vi "test-path-planner-basic.vi"() -> ()   [LabVIEW 2019]
uses:
  <vilib>/Rock Robotics/WPI/ThirdParty/MJansen/PathPlanner/PathPlannerTrajectory.ctl
  <vilib>/Rock Robotics/WPI/ThirdParty/MJansen/PathPlanner/PathPlannerState.ctl
  <vilib>/Rock Robotics/WPI/ThirdParty/JAS_Junk/TrajLib/TypeDef/ROTATION2D.ctl
  <vilib>/Rock Robotics/WPI/ThirdParty/JAS_Junk/TrajLib/TypeDef/TRAJ_STATE.ctl
  <vilib>/Rock Robotics/WPI/ThirdParty/JAS_Junk/TrajLib/TypeDef/POSE2D.ctl
  <vilib>/Rock Robotics/WPI/ThirdParty/JAS_Junk/TrajLib/TypeDef/TRANSLATION2D.ctl
  <vilib>/Rock Robotics/WPI/ThirdParty/MJansen/PathPlanner/PathPlannerWaypoint.ctl
  <vilib>/Rock Robotics/WPI/ThirdParty/JAS_Junk/TrajLib/Util_ApproxEquals.vi
  <vilib>/Rock Robotics/WPI/ThirdParty/JAS_Junk/TrajLib/TrajectoryState_Equals.vi
  <vilib>/Rock Robotics/WPI/ThirdParty/JAS_Junk/TrajLib/Pose2d_Equals.vi
  <vilib>/Rock Robotics/WPI/ThirdParty/JAS_Junk/TrajLib/Translation2d_Equals.vi
  <vilib>/Rock Robotics/WPI/ThirdParty/JAS_Junk/TrajLib/Rotation2d_Equals.vi
  <vilib>/Rock Robotics/WPI/ThirdParty/JAS_Junk/TrajLib/Util_CalcDist.vi
  <vilib>/Rock Robotics/WPI/ThirdParty/MJansen/PathPlanner/PathPlanner.lvlib
  <vilib>/Rock Robotics/WPI/ThirdParty/JAS_Junk/TrajLib/Trajectory_Library.lvlib
  <vilib>/Analysis/NI_AALBase.lvlib
panel:
  in  "Tab Control":T1(tab)
  in  "jsonReadTrajFile":string="C:\\Shares\\github\\PathPlannerLabVIEW\\PathPlannerSandbox\\PathPlannerTestPath\\Javapath1.json"
  in  "Max Velocity":dbl=3.0
  in  "Max Acceleration":dbl=2.0
  in  "stop":bool
  in  "Reversed":bool
  out "PathPlannerWayPoints":T2[](array[typedef]) {"HolonomicRotation"."SIN" format="%13.4f"; "HolonomicRotation"."COS" format="%13.4f"; "HolonomicRotation"."VALUE" format="%13.4f"; "NextControl"."Y" format="%14.3f"; "NextControl"."X" format="%14.3f"; "PrevControl"."Y" format="%14.3f"; "PrevControl"."X" format="%14.3f"; "AnchorPoint"."Y" format="%14.3f"; "AnchorPoint"."X" format="%14.3f"}
  in  "Path FileName":string="C:\\Shares\\github\\PathPlannerLabVIEW\\PathPlannerSandbox\\PathPlannerTestPath\\path1.path"
  out "LabVIEW path json read error":errorcluster
  in  "LabVIEW jsonWriteFile":string="C:\\Shares\\github\\PathPlannerLabVIEW\\PathPlannerSandbox\\PathPlannerTestPath\\LabVIEWpath1.json"
  out "Java File Read Error":errorcluster
  out "LabView Write\nJSON Error":errorcluster
  out "PathPlannerTrajectory":T5 {"States"."HolonomicAngular\nvelocity Deg/Sec"."SIN" format="%13.4f"; "States"."HolonomicAngular\nvelocity Deg/Sec"."COS" format="%13.4f"; "States"."HolonomicAngular\nvelocity Deg/Sec"."VALUE" format="%13.4f"; "States"."HolonomicRotation"."SIN" format="%13.4f"; "States"."HolonomicRotation"."COS" format="%13.4f"; "States"."HolonomicRotation"."VALUE" format="%13.4f"; "States"."AngularVelocity"."SIN" format="%13.4f"; "States"."AngularVelocity"."COS" format="%13.4f"; "States"."AngularVelocity"."VALUE" format="%13.4f"; "States"."TrajectoryState"."POSE"."ROTATION"."SIN" format="%13.4f"; "States"."TrajectoryState"."POSE"."ROTATION"."COS" format="%13.4f"; "States"."TrajectoryState"."POSE"."ROTATION"."VALUE" format="%13.4f"; "States"."TrajectoryState"."POSE"."TRANSLATION"."Y" format="%14.3f"; "States"."TrajectoryState"."POSE"."TRANSLATION"."X" format="%14.3f"; "States"."AngularAcceleration"."SIN" format="%13.4f"; "States"."AngularAcceleration"."COS" format="%13.4f"; "States"."AngularAcceleration"."VALUE" format="%13.4f"}
  out "outPathPlannerStates":T6[](array[typedef]) {"HolonomicAngular\nvelocity Deg/Sec"."SIN" format="%13.4f"; "HolonomicAngular\nvelocity Deg/Sec"."COS" format="%13.4f"; "HolonomicAngular\nvelocity Deg/Sec"."VALUE" format="%13.4f"; "HolonomicRotation"."SIN" format="%13.4f"; "HolonomicRotation"."COS" format="%13.4f"; "HolonomicRotation"."VALUE" format="%13.4f"; "AngularVelocity"."SIN" format="%13.4f"; "AngularVelocity"."COS" format="%13.4f"; "AngularVelocity"."VALUE" format="%13.4f"; "TrajectoryState"."POSE"."ROTATION"."SIN" format="%13.4f"; "TrajectoryState"."POSE"."ROTATION"."COS" format="%13.4f"; "TrajectoryState"."POSE"."ROTATION"."VALUE" format="%13.4f"; "TrajectoryState"."POSE"."TRANSLATION"."Y" format="%14.3f"; "TrajectoryState"."POSE"."TRANSLATION"."X" format="%14.3f"; "AngularAcceleration"."SIN" format="%13.4f"; "AngularAcceleration"."COS" format="%13.4f"; "AngularAcceleration"."VALUE" format="%13.4f"}
  in  "Down Button":bool
  in  "Up Button":bool
  in  "index":i32 step=20
  out "Java_TotalTime_Sec":dbl
  out "LabVIEW_TotalTime_Sec":dbl
  out "Jave and LabVIEW \nexactly equal":bool
  out "JavaStateCount":i32
  out "LabVIEWStateCount":i32
  out "States Check":bool[](array[boolean])
  out "JavaStates":T7[](array[typedef]) {"POSE"."ROTATION"."SIN" format="%13.4f"; "POSE"."ROTATION"."COS" format="%13.4f"; "POSE"."ROTATION"."VALUE" format="%13.4f"; "POSE"."TRANSLATION"."Y" format="%14.3f"; "POSE"."TRANSLATION"."X" format="%14.3f"}
  out "LabVIEWStates":T7[](array[typedef]) {"POSE"."ROTATION"."SIN" format="%13.4f"; "POSE"."ROTATION"."COS" format="%13.4f"; "POSE"."ROTATION"."VALUE" format="%13.4f"; "POSE"."TRANSLATION"."Y" format="%14.3f"; "POSE"."TRANSLATION"."X" format="%14.3f"}
  out "Differences":T7[](array[typedef]) {"POSE"."ROTATION"."SIN" format="%13.4f"; "POSE"."ROTATION"."COS" format="%13.4f"; "POSE"."ROTATION"."VALUE" format="%13.4f"; "POSE"."TRANSLATION"."Y" format="%14.3f"; "POSE"."TRANSLATION"."X" format="%14.3f"}
  out "max time diff":dbl
  out "max vel diff":dbl
  out "max accel diff":dbl
  out "max x diff":dbl
  out "max y diff":dbl
  out "max rot diff rad":dbl
  out "max curvature diff":dbl
  out "vel mean":dbl format="%0.6f"
  out "vel std dev":dbl format="%0.6f"
  out "accel mean":dbl format="%0.6f"
  out "accel std dev":dbl format="%0.6f"
  out "Java and LabVIEW \nwithin tolerance":bool
  in  "Tolerance":T7={"TimeSeconds"=0.15, "Velocity"=0.25, "Acceleration"=2.5, "POSE"={"TRANSLATION"={"X"=0.015, "Y"=0.015}, "ROTATION"={"VALUE"=0.01, "COS"=0.0, "SIN"=0.0}}, "Curvature"=1.4} {"POSE"."ROTATION"."SIN" format="%13.4f"; "POSE"."ROTATION"."COS" format="%13.4f"; "POSE"."ROTATION"."VALUE" format="%13.4f"; "POSE"."TRANSLATION"."Y" format="%14.3f"; "POSE"."TRANSLATION"."X" format="%14.3f"}
  out "XY SPLINE":cluster{dbl[], dbl[]}[](graph)
  out "XY Graph":cluster{dbl[], dbl[]}[](graph)
  out "Sample Graph":dbl[][](graph)
  out "LabVIEW Time Plot":cluster{dbl[], dbl[]}[](graph)
  out "Java Time Plot":cluster{dbl[], dbl[]}[](graph)
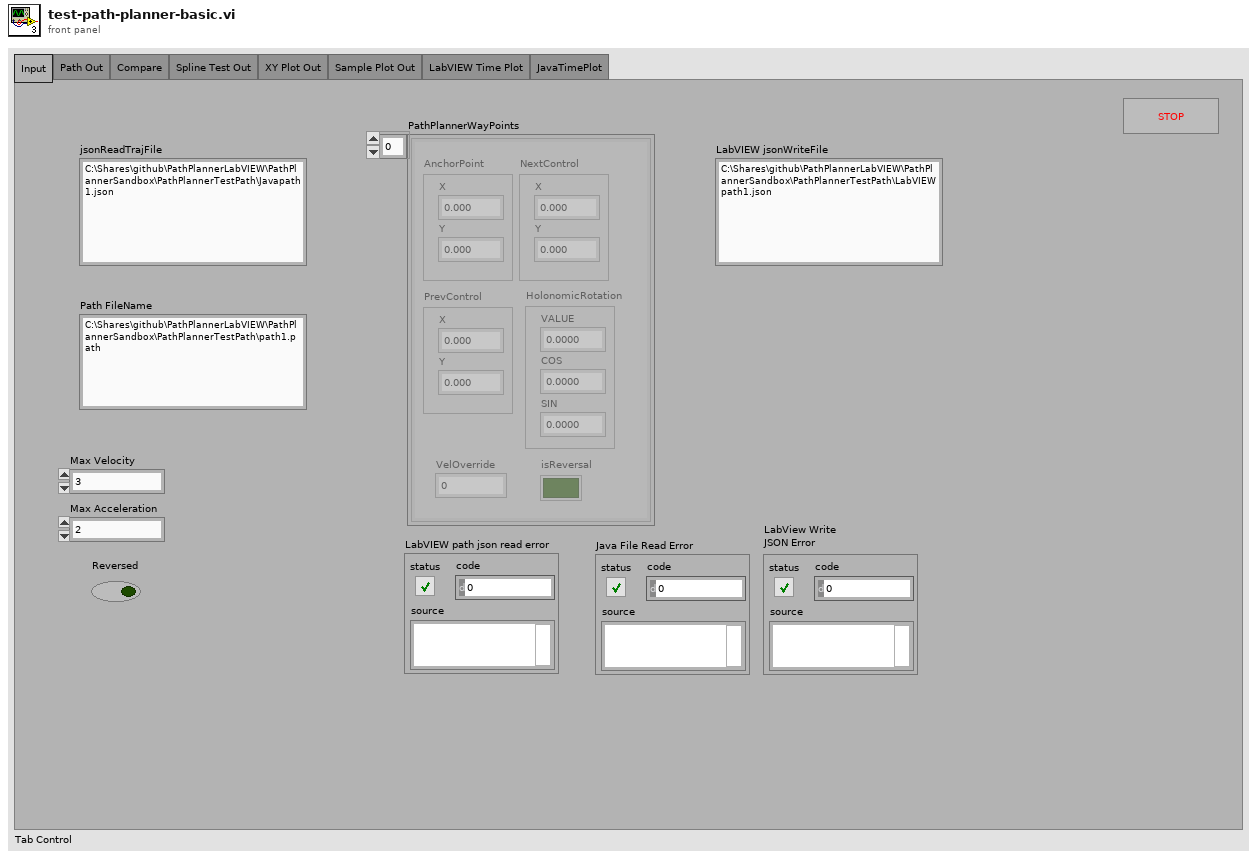
[diagram p1: front panel]
types:
  T1 = enum32{"Input", "Path Out", "Compare", "Spline Test Out", "XY Plot Out", "Sample Plot Out", "LabVIEW Time Plot", "JavaTimePlot"}
  T2 = typedef "PathPlanner.lvlib/PathPlannerWaypoint.ctl" = cluster{"AnchorPoint":T3, "PrevControl":T3, "NextControl":T3, "HolonomicRotation":T4, "VelOverride":dbl, "isReversal":bool}
  T3 = typedef "Trajectory_Library.lvlib/TRANSLATION2D.ctl" = cluster{"X":dbl, "Y":dbl}
  T4 = typedef "Trajectory_Library.lvlib/ROTATION2D.ctl" = cluster{"VALUE":dbl, "COS":dbl, "SIN":dbl}
  T5 = typedef "PathPlanner.lvlib/PathPlannerTrajectory.ctl" = cluster{"TotalTimeSeconds":dbl, "States":T6[]}
  T6 = typedef "PathPlanner.lvlib/PathPlannerState.ctl" = cluster{"AngularAcceleration":T4, "PositionMeters":dbl, "TrajectoryState":T7, "AngularVelocity":T4, "HolonomicRotation":T4, "CurveRadius":dbl, "DeltaPos":dbl, "HolonomicAngular\nvelocity Deg/Sec":T4}
  T7 = typedef "Trajectory_Library.lvlib/TRAJ_STATE.ctl" = cluster{"TimeSeconds":dbl, "Velocity":dbl, "Acceleration":dbl, "POSE":T8, "Curvature":dbl}
  T8 = typedef "Trajectory_Library.lvlib/POSE2D.ctl" = cluster{"TRANSLATION":T3, "ROTATION":T4}
  T9 = typedef "Trajectory_Library.lvlib/TRAJECTORY.ctl" = cluster{"TotalTImeSecs":dbl, "States":T7[]}
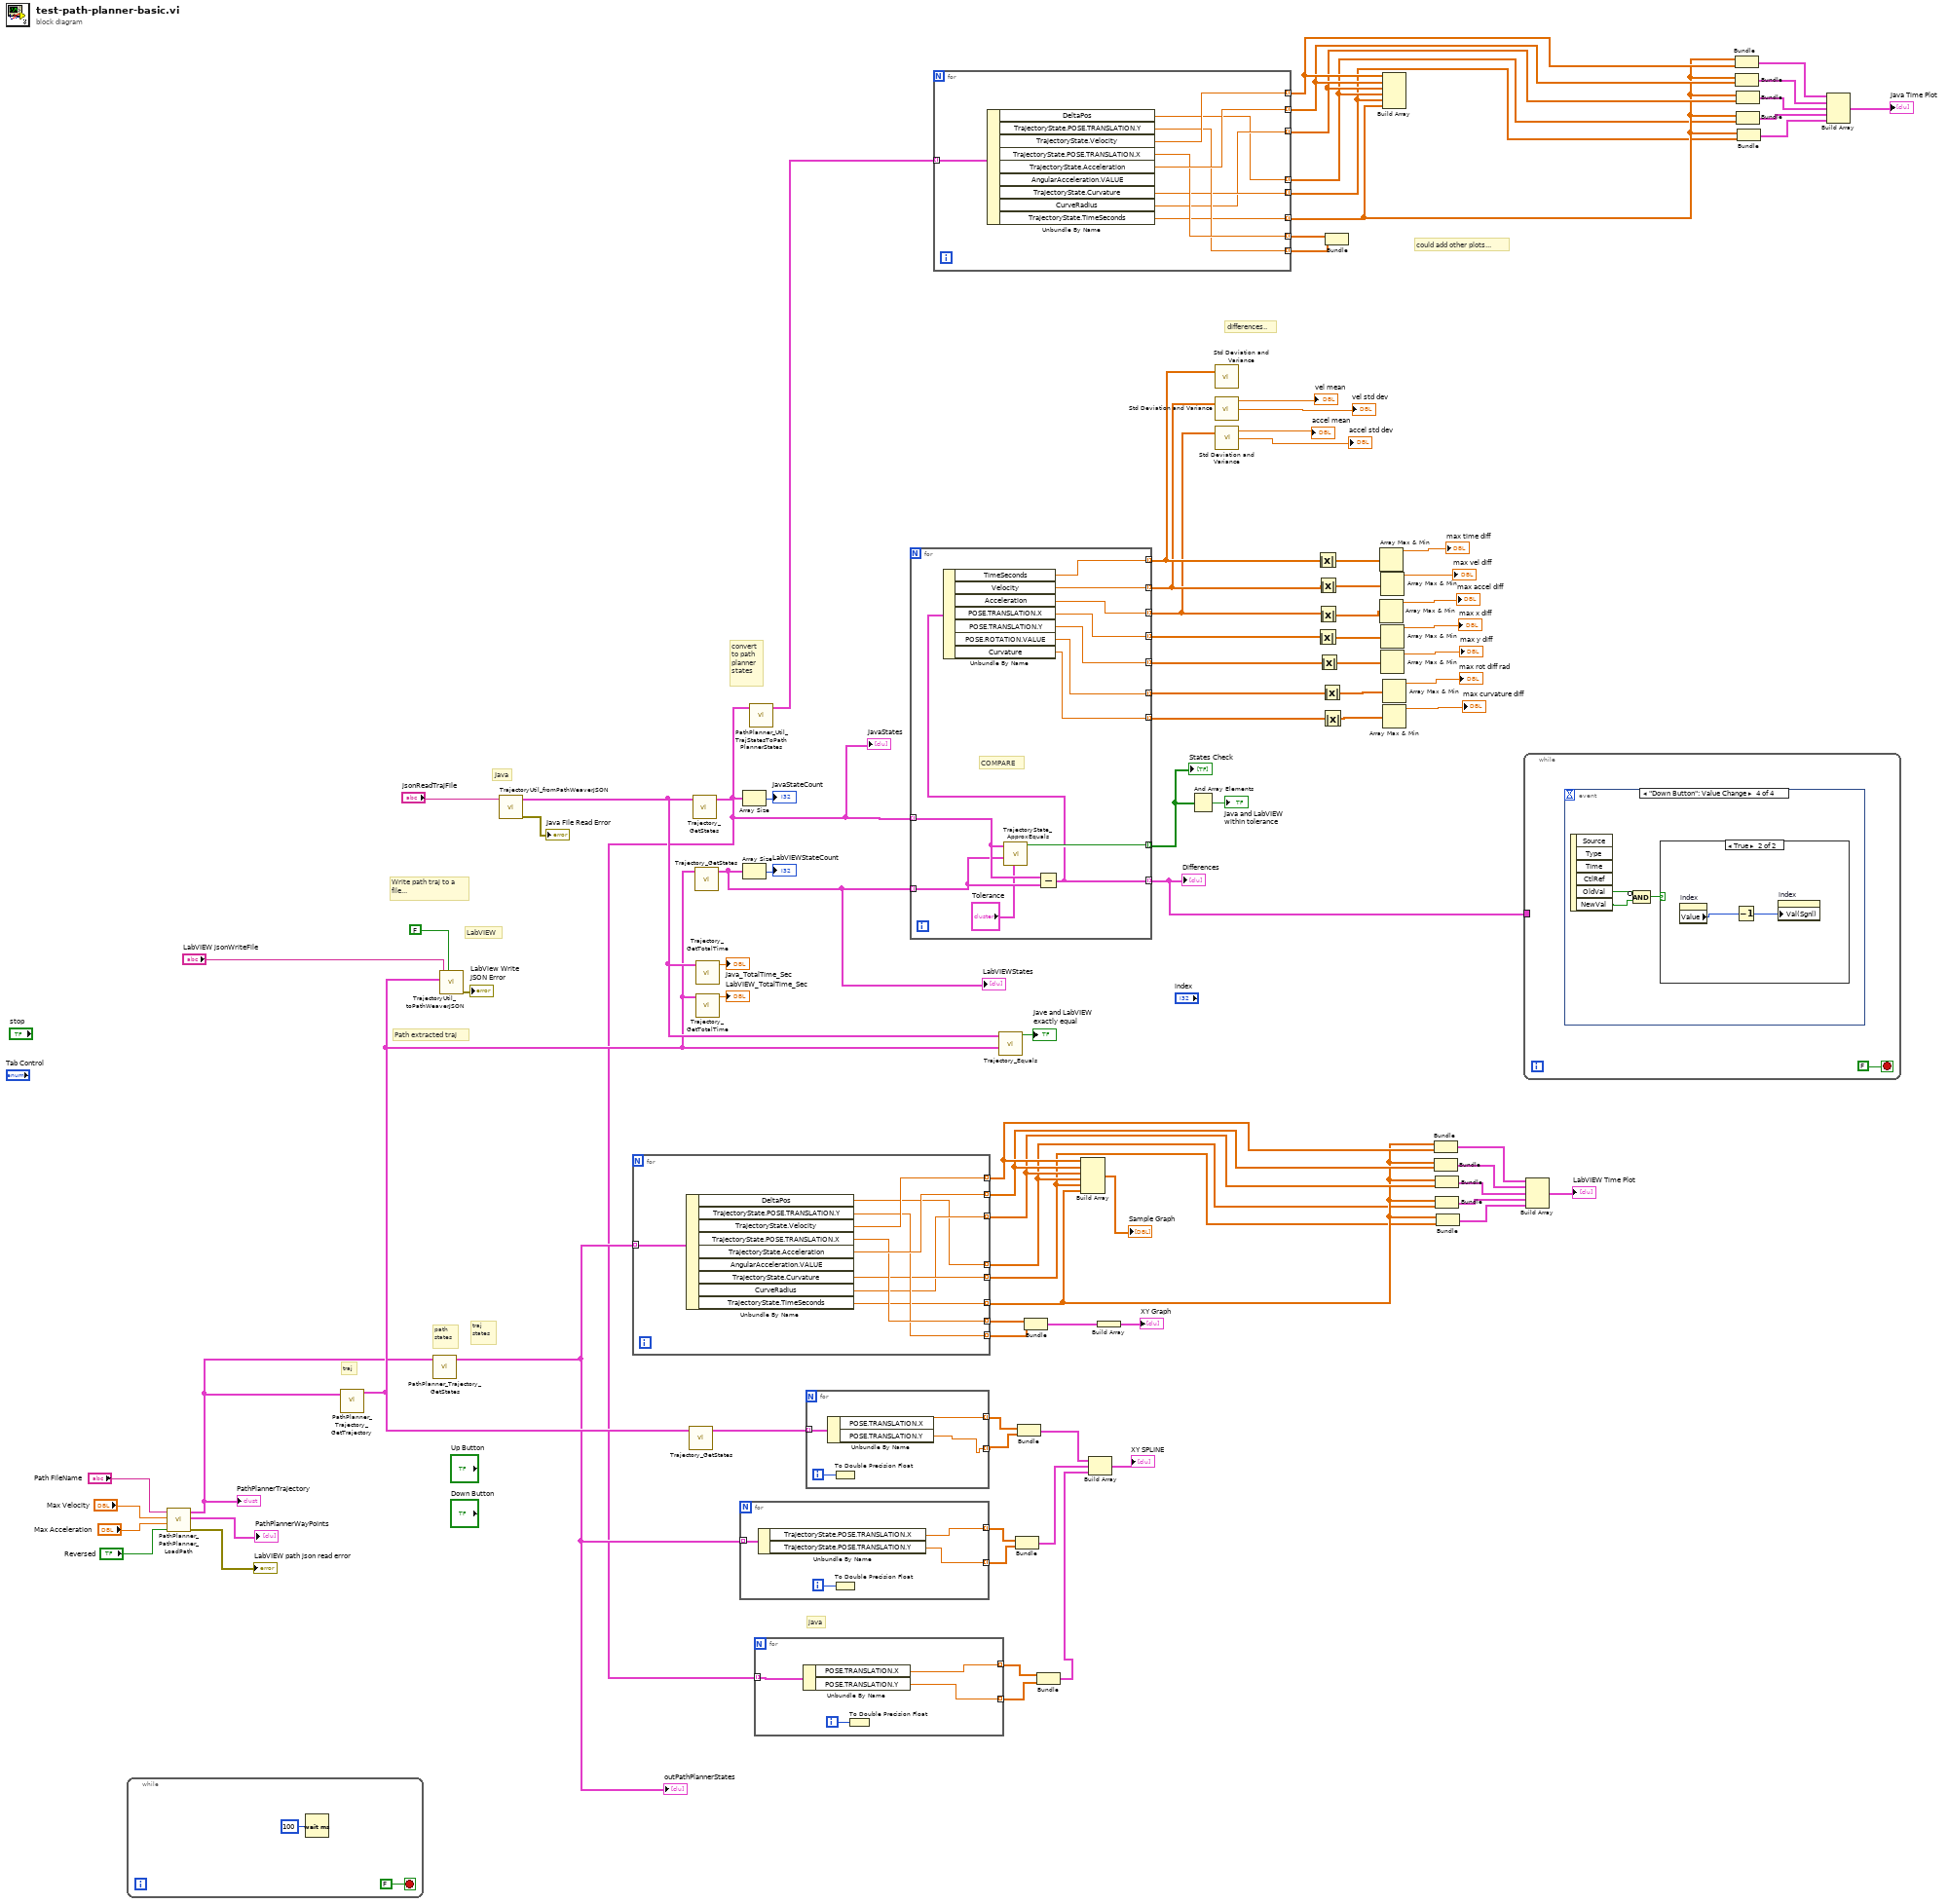
[diagram p0: block diagram]
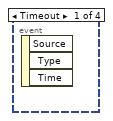
[diagram p2: hidden frame]
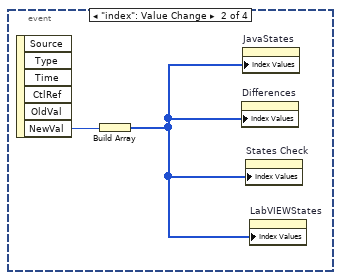
[diagram p3: hidden frame]
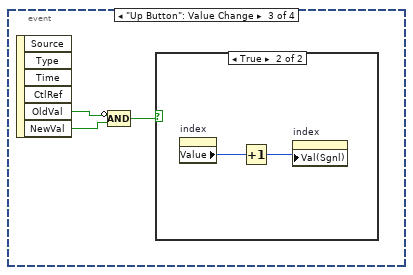
[diagram p4: hidden frame]
diagram:
  # "Write path traj to a \nfile..."
  # "Path extracted traj"
  # "traj"
  # "traj\nstates"
  # "path\nstates"
  # "differences.."
  # "could add other plots..."
  # "convert\nto path\nplanner\nstates"
  # "java"
  # "LabVIEW"
  # "Java"
  n1 = while {
    stop <- FALSE stop-if-true
    n2 = Wait (ms)(milliseconds to wait=u32 100) -> ()  [unwired: 1 out]
  }
  n3 = call <vilib>:"PathPlanner_PathPlanner_LoadPath.vi"("Reversed"="Reversed", "MaxAcceleration"="Max Acceleration", "MaxVelocity"="Max Velocity", "FileName"="Path FileName") -> ("error out"=→"LabVIEW path json read error":errorcluster, "PathPlannerWayPoints"=→"PathPlannerWayPoints":T2[], "PathPlannerTrajectory"=w63:T5)  [unwired: 4 in, 1 out]
  "PathPlannerTrajectory" <- w63
  n4 = call <vilib>:"PathPlanner_Trajectory_GetTrajectory.vi"("PathPlannerTrajectory"=w63) -> ("TRAJECTORY"=w68:T9)  [unwired: 10 in]
  n5 = call <vilib>:"PathPlanner_Trajectory_GetStates.vi"("PathPlannerTrajectory"=w63) -> ("PathPlannerStates"=w59:T6[])  [unwired: 10 in]
  "outPathPlannerStates" <- w59
  n6 = call <vilib>:"TrajectoryUtil_toPathWeaverJSON.vi"("AlwaysOverWrite"=FALSE, "inTRAJECTORY"=w68, "FileName"="LabVIEW jsonWriteFile") -> ("error out"=→"LabView Write\nJSON Error":errorcluster)  [unwired: 7 in, 1 out]
  n7 = call <vilib>:"TrajectoryUtil_fromPathWeaverJSON.vi"("FileName"="jsonReadTrajFile") -> ("error out"=→"Java File Read Error":errorcluster, "outTRAJECTORY"=w69:T9)  [unwired: 8 in, 1 out]
  n8 = for {
    tunnel: [w104] -> w32 mode=indexing
    tunnel: [w103] -> w31 mode=indexing
    tunnel: [w97] -> w28 mode=indexing
    tunnel: [w102] -> w92 mode=indexing
    tunnel: [w101] -> w91 mode=indexing
    tunnel: w59 -> [w100] mode=indexing
    tunnel: [w99] -> w27 mode=indexing
    tunnel: [w98] -> w30 mode=indexing
    tunnel: [w96] -> w29 mode=indexing
    n9 = Unbundle By Name(w100) -> ("DeltaPos"=w97:dbl, "TrajectoryState.POSE.TRANSLATION.Y"=w101:dbl, "TrajectoryState.Velocity"=w104:dbl, "TrajectoryState.POSE.TRANSLATION.X"=w102:dbl, "TrajectoryState.Acceleration"=w103:dbl, "TrajectoryState.Curvature"=w99:dbl, "CurveRadius"=w98:dbl, "TrajectoryState.TimeSeconds"=w96:dbl)  [unwired: 1 out]
  }
  n10 = call <vilib>:"Trajectory_GetStates.vi"("TRAJECTORY"=w68) -> ("States"=w73:T7[])  [unwired: 10 in]
  n11 = call <vilib>:"Trajectory_GetStates.vi"("TRAJECTORY"=w69) -> ("States"=w8:T7[])  [unwired: 10 in]
  "JavaStates" <- w8
  n12 = call <vilib>:"Trajectory_GetStates.vi"("TRAJECTORY"=w68) -> ("States"=w65:T7[])  [unwired: 10 in]
  "LabVIEWStates" <- w65
  n13 = call <vilib>:"Trajectory_GetTotalTime.vi"("TRAJECTORY"=w69) -> ("TotalTime_Sec"=→"Java_TotalTime_Sec":dbl)  [unwired: 10 in]
  n14 = call <vilib>:"Trajectory_GetTotalTime.vi"("TRAJECTORY"=w68) -> ("TotalTime_Sec"=→"LabVIEW_TotalTime_Sec":dbl)  [unwired: 10 in]
  n15 = for {
    tunnel: [w107] -> w86 mode=indexing
    tunnel: w59 -> [w106] mode=indexing
    tunnel: [w105] -> w85 mode=indexing
    i -> [w108]
    n16 = Unbundle By Name(w106) -> ("TrajectoryState.POSE.TRANSLATION.X"=w107:dbl, "TrajectoryState.POSE.TRANSLATION.Y"=w105:dbl)
    n17 = To Double Precision Float(number=w108) -> ()  [unwired: 1 out]
  }
  n18 = Array Size(array=w8) -> (size(s)=→"JavaStateCount":i32)
  n19 = Array Size(array=w65) -> (size(s)=→"LabVIEWStateCount":i32)
  n20 = call "PathPlanner_Util_TrajStatesToPathPlannerStates.vi"("TrajStates"=w8) -> ("PathPlannerStates"=w7:T6[])  [unwired: 10 in]
  n21 = for {
    tunnel: [w111] -> w81 mode=indexing
    tunnel: w8 -> [w110] mode=indexing
    tunnel: [w109] -> w80 mode=indexing
    i -> [w112]
    n22 = Unbundle By Name(w110) -> ("POSE.TRANSLATION.X"=w111:dbl, "POSE.TRANSLATION.Y"=w109:dbl)
    n23 = To Double Precision Float(number=w112) -> ()  [unwired: 1 out]
  }
  n24 = for {
    tunnel: [w115] -> w88 mode=indexing
    tunnel: [w114] -> w87 mode=indexing
    tunnel: w73 -> [w113] mode=indexing
    i -> [w116]
    n25 = Unbundle By Name(w113) -> ("POSE.TRANSLATION.X"=w115:dbl, "POSE.TRANSLATION.Y"=w114:dbl)
    n26 = To Double Precision Float(number=w116) -> ()  [unwired: 1 out]
  }
  n27 = for {
    tunnel: w8 -> [w127] mode=indexing
    tunnel: w65 -> [w126] mode=indexing
    tunnel: [w128] -> w6 mode=indexing
    tunnel: [w125] -> w64 mode=indexing
    tunnel: [w124] -> w40 mode=indexing
    tunnel: [w123] -> w39 mode=indexing
    tunnel: [w122] -> w38 mode=indexing
    tunnel: [w121] -> w55 mode=indexing
    tunnel: [w120] -> w56 mode=indexing
    tunnel: [w119] -> w57 mode=indexing
    tunnel: [w118] -> w58 mode=indexing
    # "COMPARE"
    n28 = call "TrajectoryState_ApproxEquals.vi"("Tolerance"="Tolerance", "Other TRAJ_STATE"=w126, "TRAJ_STATE"=w127) -> ("Equals"=w128:bool)  [unwired: 8 in]
    n29 = Subtract(x=w127, y=w126) -> (x-y=w125:T7)
    n30 = Unbundle By Name(w125) -> ("TimeSeconds"=w124:dbl, "Velocity"=w123:dbl, "Acceleration"=w122:dbl, "POSE.TRANSLATION.X"=w121:dbl, "POSE.TRANSLATION.Y"=w120:dbl, "POSE.ROTATION.VALUE"=w119:dbl, "Curvature"=w118:dbl)
  }
  "States Check" <- w6
  "Differences" <- w64
  n31 = for {
    tunnel: [w137] -> w19 mode=indexing
    tunnel: [w136] -> w18 mode=indexing
    tunnel: [w130] -> w15 mode=indexing
    tunnel: [w135] -> w21 mode=indexing
    tunnel: [w134] -> w20 mode=indexing
    tunnel: w7 -> [w133] mode=indexing
    tunnel: [w132] -> w14 mode=indexing
    tunnel: [w131] -> w17 mode=indexing
    tunnel: [w129] -> w16 mode=indexing
    n32 = Unbundle By Name(w133) -> ("DeltaPos"=w130:dbl, "TrajectoryState.POSE.TRANSLATION.Y"=w134:dbl, "TrajectoryState.Velocity"=w137:dbl, "TrajectoryState.POSE.TRANSLATION.X"=w135:dbl, "TrajectoryState.Acceleration"=w136:dbl, "TrajectoryState.Curvature"=w132:dbl, "CurveRadius"=w131:dbl, "TrajectoryState.TimeSeconds"=w129:dbl)  [unwired: 1 out]
  }
  n33 = call <vilib>:"Trajectory_Equals.vi"("other TRAJECTORY"=w68, "TRAJECTORY"=w69) -> ("Equals"=→"Jave and LabVIEW \nexactly equal":bool)  [unwired: 9 in]
  n34 = Bundle(w86, w85) -> (w83:cluster{dbl[], dbl[]})  [unwired: 1 in]
  n35 = Bundle(w88, w87) -> (w84:cluster{dbl[], dbl[]})  [unwired: 1 in]
  n36 = Bundle(w92, w91) -> (w90:cluster{dbl[], dbl[]})  [unwired: 1 in]
  n37 = Bundle(w81, w80) -> (w79:cluster{dbl[], dbl[]})  [unwired: 1 in]
  n38 = Build Array(w32, w31, w30, w28, w27, w29) -> (→"Sample Graph":dbl[][])
  n39 = Build Array(w84, w83, w79) -> (→"XY SPLINE":cluster{dbl[], dbl[]}[])
  n40 = Build Array(w90) -> (→"XY Graph":cluster{dbl[], dbl[]}[])
  n41 = And Array Elements(Boolean array=w6) -> (logical AND=→"Java and LabVIEW \nwithin tolerance":bool)
  n42 = call <vilib>:"Std Deviation and Variance.vi"("X"=w40) -> ()  [unwired: 1 in, 3 out]
  n43 = call <vilib>:"Std Deviation and Variance.vi"("X"=w39) -> ("mean"=→"vel mean":dbl, "standard deviation"=→"vel std dev":dbl)  [unwired: 1 in, 1 out]
  n44 = call <vilib>:"Std Deviation and Variance.vi"("X"=w38) -> ("mean"=→"accel mean":dbl, "standard deviation"=→"accel std dev":dbl)  [unwired: 1 in, 1 out]
  n45 = Absolute Value(x=w40) -> (abs(x)=w48:dbl[])
  n46 = Absolute Value(x=w55) -> (abs(x)=w51:dbl[])
  n47 = Absolute Value(x=w39) -> (abs(x)=w49:dbl[])
  n48 = Absolute Value(x=w38) -> (abs(x)=w50:dbl[])
  n49 = Absolute Value(x=w56) -> (abs(x)=w52:dbl[])
  n50 = Absolute Value(x=w57) -> (abs(x)=w53:dbl[])
  n51 = Absolute Value(x=w58) -> (abs(x)=w54:dbl[])
  n52 = Bundle(w21, w20) -> ()  [unwired: 1 in, 1 out]
  n53 = Array Max & Min(array=w48) -> (max value=→"max time diff":dbl)  [unwired: 3 out]
  n54 = Array Max & Min(array=w50) -> (max value=→"max accel diff":dbl)  [unwired: 3 out]
  n55 = Array Max & Min(array=w49) -> (max value=→"max vel diff":dbl)  [unwired: 3 out]
  n56 = Array Max & Min(array=w51) -> (max value=→"max x diff":dbl)  [unwired: 3 out]
  n57 = Array Max & Min(array=w52) -> (max value=→"max y diff":dbl)  [unwired: 3 out]
  n58 = Build Array(w19, w18, w17, w15, w14, w16) -> ()  [unwired: 1 out]
  n59 = Array Max & Min(array=w53) -> (max value=→"max rot diff rad":dbl)  [unwired: 3 out]
  n60 = Array Max & Min(array=w54) -> (max value=→"max curvature diff":dbl)  [unwired: 3 out]
  n61 = Bundle(w29, w32) -> (w26:cluster{dbl[], dbl[]})  [unwired: 1 in]
  n62 = Bundle(w29, w31) -> (w25:cluster{dbl[], dbl[]})  [unwired: 1 in]
  n63 = Bundle(w29, w30) -> (w24:cluster{dbl[], dbl[]})  [unwired: 1 in]
  n64 = Bundle(w29, w28) -> (w23:cluster{dbl[], dbl[]})  [unwired: 1 in]
  n65 = Bundle(w29, w27) -> (w22:cluster{dbl[], dbl[]})  [unwired: 1 in]
  n66 = while {
    tunnel: w64 -> [_]
    stop <- FALSE stop-if-true
    n67 = event shown="[3] \"Down Button\": Value Change" {
      selector: _ -> [_ _ _ _]
      dyn-events: _ -> [_ _ _ _]
      timeout: _ -> [_ _ _ _]
      event Timeout {
        n68 = event-data() -> ()  [unwired: 1 in, 3 out]
      }
      event "index": Value Change {
        n69 = event-data() -> ("NewVal"=w140:i32)  [unwired: 1 in, 5 out]
        n70 = Build Array(w140) -> (w139:i32[])
        n71 = property on="Differences" class="Arr (strict)"("Index Values"=w139) -> ()  [unwired: 2 in, 2 out]
        n72 = property on="JavaStates" class="Arr (strict)"("Index Values"=w139) -> ()  [unwired: 2 in, 2 out]
        n73 = property on="States Check" class="Arr (strict)"("Index Values"=w139) -> ()  [unwired: 2 in, 2 out]
        n74 = property on="LabVIEWStates" class="Arr (strict)"("Index Values"=w139) -> ()  [unwired: 2 in, 2 out]
      }
      event "Up Button": Value Change {
        n75 = event-data() -> ("OldVal"=w143:bool, "NewVal"=w142:bool)  [unwired: 1 in, 4 out]
        n76 = Compound Arithmetic op=AND(invert w143, w142) -> (w141:bool)
        n77 = case shown="True" w141 {
          frame False {
          }
          frame True {
            n78 = property on="index" class="DigNum (strict)"() -> ("Value"=w144:i32)  [unwired: 2 in, 2 out]
            n79 = Increment(x=w144) -> (x+1=w145:i32)
            n80 = property on="index" class="DigNum (strict)"("Val(Sgnl)"=w145) -> ()  [unwired: 2 in, 2 out]
          }
        }
      }
      event "Down Button": Value Change {
        n81 = event-data() -> ("OldVal"=w147:bool, "NewVal"=w146:bool)  [unwired: 1 in, 4 out]
        n82 = Compound Arithmetic op=AND(invert w147, w146) -> (w148:bool)
        n83 = case shown="True" w148 {
          frame False {
          }
          frame True {
            n84 = property on="index" class="DigNum (strict)"() -> ("Value"=w149:i32)  [unwired: 2 in, 2 out]
            n85 = Decrement(x=w149) -> (x-1=w150:i32)
            n86 = property on="index" class="DigNum (strict)"("Val(Sgnl)"=w150) -> ()  [unwired: 2 in, 2 out]
          }
        }
      }
    }
  }
  n87 = Build Array(w26, w25, w24, w23, w22) -> (→"LabVIEW Time Plot":cluster{dbl[], dbl[]}[])
  n88 = Bundle(w16, w19) -> (w13:cluster{dbl[], dbl[]})  [unwired: 1 in]
  n89 = Bundle(w16, w18) -> (w12:cluster{dbl[], dbl[]})  [unwired: 1 in]
  n90 = Bundle(w16, w17) -> (w11:cluster{dbl[], dbl[]})  [unwired: 1 in]
  n91 = Bundle(w16, w15) -> (w10:cluster{dbl[], dbl[]})  [unwired: 1 in]
  n92 = Bundle(w16, w14) -> (w9:cluster{dbl[], dbl[]})  [unwired: 1 in]
  n93 = Build Array(w13, w12, w11, w10, w9) -> (→"Java Time Plot":cluster{dbl[], dbl[]}[])
